vi "XYZ mov setup unbundler-DBL.vi"(8 "error in (no error)":errorcluster, 9 "Keys Array":T1, 10 "Section":string, 11 "User profile ref":T2) -> (0 "error out":errorcluster, 3 "User profile ref":T2)   [LabVIEW 2017]
uses:
  <vilib>/Utility/config.llb/Config Data RefNum.ctl
  Typedefs/Ini file interface (DBL).ctl
  User Interface/Windows/Position control window/Globals/Pos ctrl window globals.vi
  <vilib>/Utility/config.llb/NI_LVConfig.lvlib
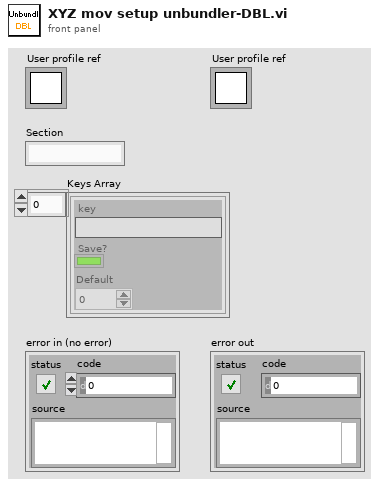
[diagram p1: front panel]
types:
  T1 = typedef "Ini file interface (DBL).ctl" = cluster{"key":string, "Save?":bool, "Default":dbl}[]
  T2 = typedef "NI_LVConfig.lvlib/Config Data RefNum.ctl" = refnum<k1>
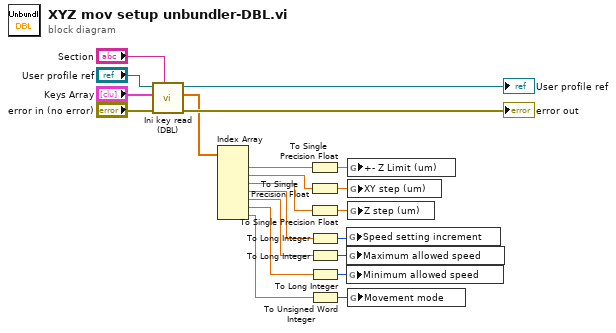
[diagram p0: block diagram]
diagram:
  n1 = call "Ini key read (DBL).vi"("Section name"="Section", "error in (no error)"="error in (no error)", "Parameter names & setup"="Keys Array", "Ini file refnum in"="User profile ref") -> ("error out"=→"error out":errorcluster, "Value read/used"=w1:dbl[], "Ini file refnum out"=→"User profile ref":T2)  [unwired: 5 in]
  n2 = Index Array(array=w1) -> (element #1=w10:dbl, element #2=w12:dbl, element #3=w14:dbl, element #4=w8:dbl, element #5=w7:dbl, element #6=w6:dbl, element #7=w5:dbl)  [unwired: 7 in]
  n3 = To Single Precision Float(number=w10) -> (single precision float=w11:sgl)
  n4 = To Single Precision Float(number=w12) -> (single precision float=w13:sgl)
  n5 = To Single Precision Float(number=w14) -> (single precision float=w15:sgl)
  n6 = To Long Integer(number=w8) -> (32bit integer=w4:i32)
  n7 = To Long Integer(number=w7) -> (32bit integer=w3:i32)
  n8 = To Long Integer(number=w6) -> (32bit integer=w2:i32)
  n9 = To Unsigned Word Integer(number=w5) -> (unsigned 16bit integer=w9:u16)
  n10 = global write "Pos ctrl window globals.vi" "Speed setting increment"(w4) -> ()
  n11 = global write "Pos ctrl window globals.vi" "Maximum allowed speed"(w3) -> ()
  n12 = global write "Pos ctrl window globals.vi" "Minimum allowed speed"(w2) -> ()
  n13 = global write "Pos ctrl window globals.vi" "+- Z Limit (um)"(w11) -> ()
  n14 = global write "Pos ctrl window globals.vi" "XY step (um)"(w13) -> ()
  n15 = global write "Pos ctrl window globals.vi" "Z step (um)"(w15) -> ()
  n16 = global write "Pos ctrl window globals.vi" "Movement mode"(w9) -> ()
